vi "write_params.vi"(8 "error in (no error)":errorcluster caption="entrée d'erreur (pas d'erreur)", 10 "params":T1={"penalty"="l2", "dual"=FALSE, "tol"=0.0001, "C"=1.0, "fit_intercept"=TRUE, "intercept_scaling"=1.0, "class_weight"={"class_weight_type"="None", "class_weight_dict"=""}, "random_state"=0.0, "solver"="lbfgs", "max_iter"=100.0, "multi_class"="auto", "verbose"=0.0, "warm_start"=FALSE, "n_jobs"=1.0, "l1_ratio"={"l1_ratio_type"="None", "l1_ratio_float"=0.0}}, 11 "LogisticRegression en entrée":refnum<class "LogisticRegression.lvclass">) -> (0 "error out":errorcluster caption="sortie d'erreur", 3 "LogisticRegression en sortie":refnum<class "LogisticRegression.lvclass">)   [LabVIEW 2020, in "LogisticRegression.lvclass"]
uses:
  LogisticRegression.lvclass
  Controls/logistic_regression_params.ctl
  LogisticRegression.lvclass/LogisticRegression.ctl
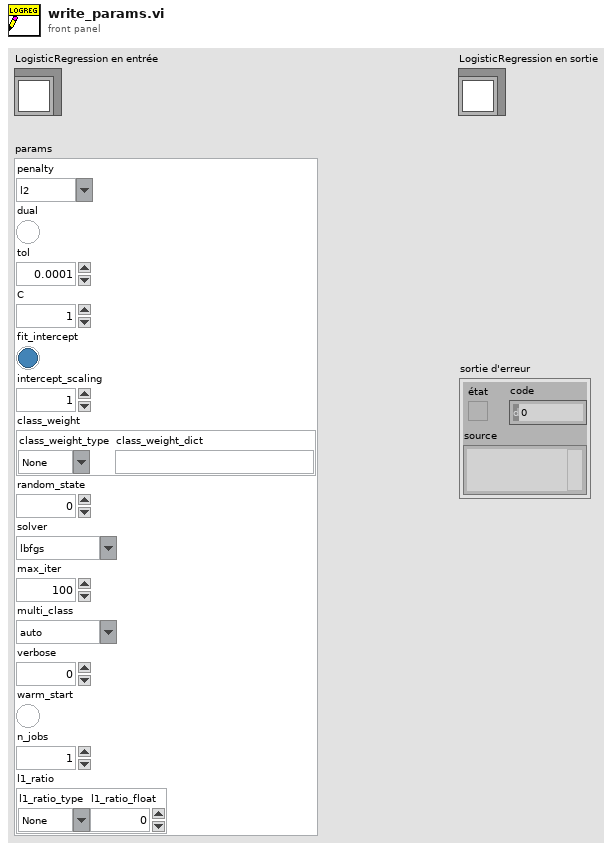
[diagram p1: front panel]
types:
  T1 = typedef "logistic_regression_params.ctl" = cluster{"penalty":string, "dual":bool, "tol":dbl, "C":dbl, "fit_intercept":bool, "intercept_scaling":dbl, "class_weight":cluster{"class_weight_type":string, "class_weight_dict":string}, "random_state":dbl, "solver":string, "max_iter":dbl, "multi_class":string, "verbose":dbl, "warm_start":bool, "n_jobs":dbl, "l1_ratio":cluster{"l1_ratio_type":string, "l1_ratio_float":dbl}}
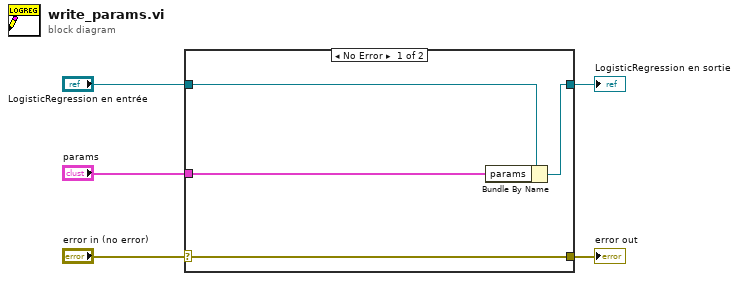
[diagram p0: block diagram]
diagram:
  n1 = case shown="No Error" "error in (no error)" {
    selector: "error in (no error)" -> [w9 w10]
    tunnel: [w9 w10] -> w4
    tunnel: [w7 w11] -> w2
    tunnel: "LogisticRegression en entrée" -> [w8 w11]
    tunnel: "params" -> [w6 _]
    frame No Error {
      n2 = Bundle By Name(cluster=w8, "params"=w6) -> (w7:refnum<class "LogisticRegression.lvclass">)
    }
    frame Error {
    }
  }
  "error out" <- w4
  "LogisticRegression en sortie" <- w2
